vi "Close TDMS LOG.vi"(8 "error in (no error)":errorcluster, 10 "Fault Index":i32, 11 "Refnum in":refnum<k34>) -> (0 "error out":errorcluster, 3 "Refnum out":refnum<k34>)   [LabVIEW 2014]
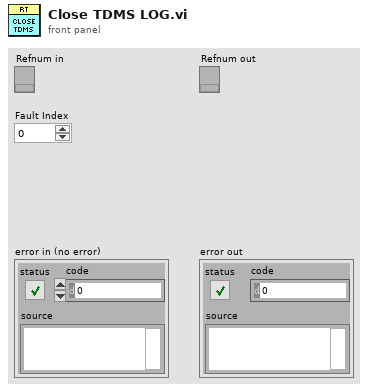
[diagram p1: front panel]
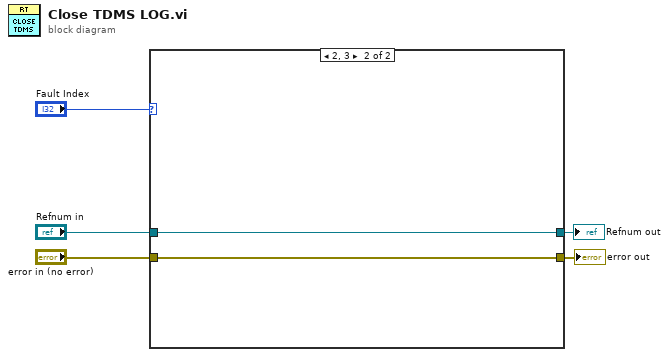
[diagram p0: block diagram]
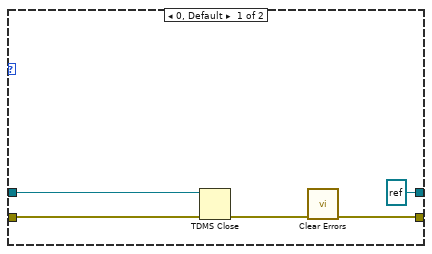
[diagram p2: hidden frame]
diagram:
  n1 = case shown="2, 3" "Fault Index" {
    tunnel: "error in (no error)" -> [w9 w12]
    tunnel: "Refnum in" -> [w10 w11]
    tunnel: [refnum<k34> refnum ("Refnum in") w11] -> w4
    tunnel: [w6 w12] -> w5
    frame 0, Default {
      n2 = TDMS Close(8:w9, 11:w10) -> (0:w8:errorcluster)  [unwired: 1 out]
      n3 = call <vilib>:"Clear Errors.vi"("error in (no error)"=w8) -> ("error out"=w6:errorcluster)  [unwired: 5 in, 1 out]
    }
    frame 2, 3 {
    }
  }
  "Refnum out" <- w4
  "error out" <- w5
